vi "claustering trial 2.vi"() -> ()   [LabVIEW 2014]
panel:
  out "x = y?":bool[](array[boolean])
  out "Array 3":string[](array[string])
  out "logical AND":bool
  in  "how many clusters":i32
  in  "wf2":string[](array[string])=["0 3 0", "0 -2 0", "0 1 0", "0 3 -2", "2 -2 0", "0 2 0", "3 -2 0", "0 -3 4", "0 4 0", "-2 0 -2", "0 -3 0", "3 -2 2", "1 -1 0", "0 2 -2", "-2 3 -2", "0 -1 0", "0 -4 0", "0 2 -2 0", "-1 0 3", "0 -2 3", "2 0 -2", "0 3 -2 0", "0 -3 4 0", "-3 0 3", "0 3 -3", "4 -3 0", "-2 0 -3", "0 -2 3 -2", "-2 2 0", "0 3 -2 2", "3 -2 2 0", "2 0 2", "3 -3 0", "2 0 3", "0 -2 0 -2", "-3 4 0", "0 3 -3 0", "-1 0 3 0", "-2 0 1", "2 -1 0", "0 -3 4 -3", "0 3 -2 2 0", "-2 0 1 0", "-3 0 4", "0 -2 2", "-2 3 -2 0", "0 3 -2 3", "0 1 -1 0", "1 0 1", "0 -3 0 3", "0 -3 3", "3 0 -3", "0 -1 0 3", "4 0 1 0", "0 -2 3 -2 0", "2 0 3 -2 0", "0 2 -1", "3 -3 0 4 0", "-2 0 -4", "-3 0 -2", "3 0 3", "0 3 0 3 0", "0 3 -2 3 -2", "-2 3 -2 2", "-3 0 1", "-2 0 3", "-2 0 -3 0", "0 3 -2 2 0 2", "2 0 2 0", "1 -1 0 3", "0 3 -2 0 -2 2", "-2 0 -2 2", "2 0 -2 3 -2", "1 0 -2", "1 0 3", "2 0 -4 0", "-1 0 1", "0 2 0 4", "4 0 -2", "0 -2 0 1", "0 -1 0 3 0", "0 2 0 3 -2 0", "0 3 -2 0 1 0", "-1 0 -1 0", "-2 2 0 -2", "2 0 -2 0 -2", "0 4 0 1 0", "0 1 0 4 0", "0 1 0 -3", "0 -3 0 3 -2", "1 0 -3 0", "4 0 -4 0 1", "-1 0 -4", "0 -3 3 -3 0 4 0", "0 -4 0 3", "0 3 0 2", "1 0 1 0", "0 4 0 3", "1 -1 0 -3 4 0", "3 -2 0 -4", "2 -1 2 0", "-4 1 0", "3 -2 0 -4 0", "-2 0 -3 4", "0 -3 4 -3 0", "0 -2 0 -3", "-2 0 -3 4 -3 0", "2 -2 3", "0 2 -1 0", "2 0 2 -2 0", "0 -3 4 0 2", "1 0 2", "-3 4 0 2 0", "-2 0 -4 1", "0 3 -2 0 -4", "0 2 0 2", "-2 3 0", "1 0 -3", "0 3 0 -3 4", "-3 4 0 2", "-2 0 -2 2 -2 0", "2 -2 0 -3 4", "0 -3 4 -3 0 3", "4 -3 0 3 0", "3 0 -2", "0 -2 0 -2 0", "4 -3 0 3", "0 4 -3 0", "-3 0 -2 0", "-1 0 -1", "1 0 4", "2 0 2 -2", "-2 0 -2 0", "0 -1 0", "0 -2 3", "3 -2 0", "-2 3 -2 0", "0 2 0", "0 1 0", "0 4 0", "2 0 -1 0", "0 3 -2", "2 -2 3", "-2 0 2", "0 2 -2 0", "4 -3 0", "-3 0 -2 0", "0 3 0", "0 -3 -2", "-2 3 -2 0 3"]
  in  "wf1":string[](array[string])=["-2 2 0", "1 -1 0", "0 1 0", "0 -1 0", "3 -3 0", "0 3 0", "0 1 -1", "0 4 0", "0 2 0", "2 -1 0", "-1 0 1", "0 -2 0", "-4 1 0", "1 0 1", "0 1 -1 0", "-1 0 -3", "-1 0 4", "0 4 0 -2", "0 4 -4", "-1 0 1 0", "0 3 -3 0", "0 -4 1", "0 4 -4 1", "-4 4 0", "-1 0 3", "0 -2 3", "0 -3 4", "1 0 1 -1", "-2 0 -3", "0 -3 0", "0 -3 3", "-2 3 -3 0", "1 0 -2", "-2 3 -2", "4 -4 1", "1 -1 0 4 -4 1", "-1 0 4 -4 1 -1", "-4 1 0 1 -1 0", "0 1 0 -4", "0 1 0 -2", "-1 0 -1 0", "2 -1 0 1", "1 -1 0 1 0", "3 -2 0", "0 -2 2", "2 0 2", "3 -3 0 1", "-3 0 3", "-2 2 0 -3", "0 3 -3", "-3 0 -4 4", "0 4 0 -2 3", "0 -4 4", "-1 0 3 0", "4 -4 1 0 4", "4 0 1 0", "1 -1 0 -3", "-2 0 1 -1", "0 4 -4 1 0", "0 -4 4 0 1", "1 0 -2 3 -2", "1 0 4", "0 -4 1 0", "0 1 0 -4 1 0", "-2 0 1", "4 -3 0", "-3 0 4", "0 4 -3 0", "1 -1 0 4 -4 1 -1 0", "4 -4 1 0", "1 0 4 0", "1 -1 0 -1 0", "0 -4 0", "4 0 1", "0 1 0 1 0", "2 0 4 0", "0 -2 0 2 0", "2 0 1", "-1 0 -3 4", "4 0 2 0", "0 -2 0 1", "-1 0 4 -4 1", "3 -2 3", "3 -2 2 0", "1 -1 0 3", "-1 0 -1", "0 -1 1", "-1 0 1 0 3", "0 -4 1 0 1 -1 0", "0 3 -2", "0 1 0 3", "1 -4 0", "0 -2 2 0", "1 -1 1 -1 0", "0 1 0 3 -3 0", "-3 0 -3 3", "0 -3 3 0", "0 3 0 -2 0", "0 2 0 2", "-4 0 -2", "3 0 3", "3 0 3 0", "0 -3 3 -2", "0 2 -2 3 -3 0", "-2 2 0 -3 3", "-3 0 1", "3 -3 0 3", "0 3 -3 0 1", "0 3 0 2", "2 0 -3", "-2 3 -3", "3 -2 2", "-4 1 -1", "2 0 -3 3", "1 -1 0", "-1 0 1", "0 1 0", "0 -1 0", "0 1 -1", "-1 0 -1", "0 4 0", "2 -1 0", "-1 0 1 -1", "-1 0 4", "0 -3 0", "0 1 -1 0", "-1 1 -1", "-1 0 -3", "-1 0 -1 0", "0 -1 0 1", "1 -1 0 -1", "-1 1 -1 0", "1 -1 1", "4 0 2", "0 1 -1 0 1", "1 -1 0 4", "0 1 0 -4", "0 4 -4", "-1 0 -1 0 1", "-1 0 4 0", "0 1 -1 1 -1 0", "1 0 -4 0", "1 0 -4", "0 4 0 -1 0", "-1 0 1 0", "0 4 -4 0", "-1 0 -3 4 0", "0 1 0 -1 0 -3", "0 1 0 -4 0", "-4 0 4", "0 -1 1 -1", "-2 2 -1 0", "0 -3 0 -1 0", "2 -1 0 -3", "-1 0 3 0", "-1 0 -3 0", "-1 0 -2", "0 2 0", "1 -1 0 4 0", "-1 0 4 0 -1 0", "0 1 -1 1 -1 0 4", "0 -2 2 -2", "-1 0 -1 0 1 0", "3 0 1 0", "0 4 0 1 -1", "1 -1 0 1", "0 1 -1 1", "1 -1 1 -1", "0 1 -1 1 -1", "1 -1 1 -1 0", "0 -1 1", "0 -4 0", "-3 0 -1", "4 0 -1", "-1 1 -1 0 4", "1 -1 1 -1 0 4"]
  in  "jon1":string[](array[string])=["0 3 0", "0 1 0", "0 2 0", "0 4 0", "0 4 -4", "0 -3 4", "0 -3 0", "0 -4 0", "0 3 -2", "0 -1 0", "-4 1 0", "1 0 3", "0 2 0 -3", "2 0 3", "3 -3 0", "-3 0 3", "0 -3 3", "0 -3 4 -3 0", "0 -2 0", "3 -2 0", "0 3 0 1 0", "0 -3 4 0", "2 -2 0", "-2 0 -3", "4 0 2", "-3 0 2", "0 3 -3 0", "4 -4 0", "0 -1 2", "3 0 4", "0 3 -2 0", "0 -3 0 3", "1 0 -1", "0 4 -4 0", "-2 0 3", "0 2 -2 0", "0 2 0 -3 4", "3 -3 0 -3", "4 0 2 0", "3 0 -2", "0 -3 3 0", "-1 0 3", "0 -1 2 0", "-4 0 -1", "2 0 3 0", "0 3 0 3", "-4 0 3", "0 4 -4 1", "4 0 -3", "0 -1 0 4", "0 3 -3 0 2", "0 -2 0 3", "0 -3 4 0 3 0", "-3 0 4 0", "0 3 0 3 0", "0 4 0 -3 0", "-3 4 0", "2 0 -3 4", "0 2 0 -3 4 0", "0 1 0 2", "0 -2 3", "-2 0 -2", "0 -3 4 0 2", "0 -3 3 0 -2 2", "1 0 -3", "0 -1 1 0", "4 -4 0 -4", "-4 0 3 0", "2 0 -3", "-2 0 3 0", "0 4 -4 1 0", "-4 1 0 -1 2 0", "3 0 4 -4", "0 -3 4 -3 0 2", "3 0 3", "-1 0 -3", "-3 4 -3", "4 -3 0", "0 -3 4 -3", "-3 4 -3 0", "4 0 2 0 3", "0 2 0 3", "-4 1 0 -4 0 4 -4", "-4 1 -1", "-1 0 -4 0", "1 0 3 -2", "0 -1 0 3", "0 3 0 4 0", "0 2 0 3 0 1 0", "-4 1 -4 1", "1 -4 1 0", "0 -4 4", "0 1 0 4", "1 -4 1", "-3 0 1", "0 4 -4 0 -1 0", "-3 0 4", "2 0 -3 4 0", "1 0 2", "4 -3 0 2", "-3 4 -3 0 2", "3 0 1", "0 3 0", "0 -3 4", "0 -3 3", "0 3 -3 0", "0 2 0", "4 -3 0", "0 3 -3", "0 3 -2", "0 -3 4 -3 0", "-4 0 -3", "3 0 -3", "0 -4 0", "-3 0 -3", "0 -3 3 0 3", "0 -3 3 0", "0 -2 0", "-3 0 3", "3 -3 0", "3 0 3", "-3 4 0", "-4 0 -3 4", "-3 0 4", "0 -1 0", "3 0 -3 3", "-3 3 0", "0 3 -2 0", "0 -3 4 0", "1 0 -3 4", "0 -3 0", "0 -1 0 -3", "-3 0 3 0", "-2 0 3 -2", "0 1 0", "0 -2 0 3", "-2 0 -3", "0 3 0 -3", "3 0 3 -3", "3 -3 0 3", "-3 0 -3 3 0", "0 -3 4 -4 0", "0 2 0 -2", "-2 0 3", "0 3 -2 3 0", "-2 3 0 -3 3", "3 0 -1", "-3 0 -4", "1 -1 0", "-4 0 -2", "0 3 -3 0 4", "-2 3 0", "-1 0 3 -2", "-3 4 -3", "0 -3 4 -3", "-3 4 -3 0", "-3 3 0 3", "-2 0 2"]
  in  "jon2":string[](array[string])=["0 3 0", "0 -1 0", "0 4 0", "-1 0 3", "0 -3 4", "0 -3 3", "1 -1 0", "0 3 -2", "0 2 0", "0 1 -1", "4 -3 0", "-4 0 -3", "0 -4 0", "4 0 2", "0 1 -1 0", "0 1 0", "0 4 -4", "3 -2 2", "2 -1 0", "0 -2 0", "0 -3 4 0", "-1 0 -3", "0 3 -2 0", "0 -3 3 -3 0", "0 -3 4 -3 0", "4 0 4", "0 1 -1 0 3", "3 -2 2 0", "-2 2 0", "3 0 1", "0 4 0 2", "0 2 -1", "2 0 4", "-1 0 4", "0 -3 3 0", "-1 0 1", "-1 0 -1 0", "-1 0 -1", "4 -3 0 2", "0 -3 0", "-4 0 -3 0", "-3 0 3 -2", "0 3 -2 2 0", "-4 0 -3 3", "0 3 0 -4", "2 0 4 -4", "0 2 0 4", "0 4 0 -4", "2 -1 0 1 -1 0", "0 2 -1 0", "-1 0 -3 3", "0 -4 4 0", "0 4 -4 0", "-4 0 3 0", "0 -2 3", "-3 0 -3", "0 -2 0 -3", "-3 0 1", "-2 3 0", "0 3 0 -2", "0 4 -3 0", "4 -3 0 2 0", "0 -3 4 -3 0 3 -2 2 0", "3 0 -3 4 -3 0", "-1 0 3 -2 3", "-1 0 3 -2", "0 1 0 3", "1 0 3", "4 -3 0 -2", "-4 0 -3 4", "-2 0 3 0", "2 0 2", "0 2 0 2 0", "-4 4 -3 0", "0 -4 0 -3", "3 0 3 0", "-4 0 -3 3 0", "4 0 3", "0 4 0 4", "4 0 4 0", "0 4 0 -4 0", "0 -1 0 -2", "4 0 2 0", "1 0 -3", "0 -4 1 -4", "0 4 -4 0 -3", "-2 2 0 4 -4", "0 4 -4 4 -4", "4 0 2 -2", "0 4 0 -2", "0 3 0 1", "4 -4 1", "4 0 2 -1 0", "0 -4 4 0 2", "-1 0 3 0", "0 3 -2 0 -1 0", "1 -1 0 4", "0 4 0 1", "-1 0 4 0", "1 0 3 -2 0 -1 0", "0 -4 0 3 0 -4", "-1 0 -4", "1 -4 0", "1 0 4 0", "0 -1 0 -1 0", "-1 0 -3 3 0", "0 -1 0 -1 0 -3", "-2 2 -1 0", "0 -1 0 3 -2", "2 -1 0 1 -1 0 3", "-2 3 -2 2 -1", "-2 2 -1", "0 -1 0 4", "3 0 1 0", "0 3 -2 0 -1 0 -1 0", "-3 4 0", "3 0 -1", "0 4 -3", "3 0 3", "-4 0 3", "4 -4 0", "0 -1 0 -1", "1 -1 0", "0 -1 0", "0 1 0", "0 1 -1 0", "0 4 0", "0 3 0", "-1 0 4", "-1 0 -3 3", "1 0 1", "-4 1 -1", "0 4 0 2", "0 -1 0 -3", "3 -2 2 -1 0", "2 -1 0", "0 1 -1", "-1 0 3", "-1 1 -1 0", "-3 0 1", "-1 0 3 0 -4", "-1 0 -3", "1 -1 0 -3 3", "1 -1 0 3", "2 -1 0 4 -4", "1 0 1 0", "0 -1 0 4", "2 0 3 0 -1", "-4 1 -1 0"]
  in  "CSS validated and checked":string[](array[string])=["0 1 0", "0 -1 0", "0 2 0", "0 4 0", "-4 1 0", "0 -4 0", "0 -2 0", "1 0 4", "1 -4 0", "0 -3 3", "0 -3 0", "1 -1 0", "-2 2 0", "0 1 -4", "2 0 -3", "0 -3 3 0", "-1 0 -1", "0 -1 1", "2 -1 0", "0 2 -1", "-3 0 1", "0 1 0 4", "1 0 4 0", "-3 3 0", "1 0 -3", "3 -2 0", "2 0 -3 0", "1 0 -1", "-4 0 -1", "0 -4 1", "2 0 -1", "0 -2 2", "-4 0 -3", "0 -1 1 0", "0 2 0 -3", "3 -3 0", "-4 0 1 0", "-4 1 -4 0", "-4 1 0 4", "0 1 -4 0", "-4 1 -4", "0 2 -1 0", "1 0 3", "0 -3 4 0", "-2 0 2", "1 0 1", "4 0 2 0", "0 2 0 3", "0 -1 2", "-1 0 -4", "1 0 -4", "0 -1 0 -1", "-1 0 2", "-1 0 -1 0", "1 0 -2", "0 -4 0 -1", "0 -2 2 0", "-1 0 1", "2 0 2", "0 1 -1 0", "0 3 -3 0", "-4 0 -2", "0 4 -4", "0 -4 0 -3", "0 4 0 1", "0 -2 0 2", "0 4 0 2 0", "-3 0 1 -4 0 -3", "2 0 1 0", "-2 0 2 0", "0 3 -2 0", "-3 3 0 -2 0", "3 -3 0 1", "-3 0 1 0", "4 -4 0", "0 4 -4 0", "0 -3 3 0 -2", "2 0 2 0", "-2 0 -1", "0 -4 0 1 0", "2 0 -4 0", "2 0 -1 0", "-1 3 -2", "2 0 1", "1 0 -3 3 0", "-4 1 -1", "-4 1 -1 0", "-1 0 -3", "3 -2 2", "-1 1 -1 0", "2 0 4", "1 0 -1 0", "0 -1 2 -1", "0 2 0 -2", "-3 0 -4 1", "0 1 0 -1", "-1 3 0", "0 -1 0 -4", "-2 0 -1 0", "4 0 4", "-4 1 0 4 0", "-4 0 -2 0", "-4 0 2", "0 -2 0 2 0", "0 2 0 -4 0", "2 0 4 0", "4 0 -2", "0 1 0 -4 0", "3 0 1", "2 -2 0", "4 0 -2 0", "0 2 0 4", "1 -4 0 1 0", "0 2 0 -2 0", "-2 2 0 -1 0", "-2 2 0 -1", "-1 0 4 0", "-2 0 4", "-4 1 0 3", "0 -3 0 1", "-2 2 0 -3 0", "0 1 0 3", "0 2 0 1", "0 1 0 1 -4", "0 1 -4 1", "-4 1 0 -3", "1 0 -3 0", "-3 0 -2", "2 -1 0 -1 0", "-3 3 0 -2", "1 0 4 -4 0", "0 -4 0 -3 0", "0 -4 0 1 0 -3 3 0", "0 -3 3 0 2 0 -3 0", "0 -3 3 -3 0", "3 -2 0 1", "-4 0 3", "-2 0 1", "0 3 0", "0 -3 4", "-3 4 0", "-3 0 4", "0 3 -3 0 1 -4 0 -3 3", "0 -2 0 -1", "-4 1 0 -2", "-4 0 -2 0 -1", "-2 0 -4", "0 1 0 -2", "0 -1 0 2 0", "0 -2 2 0 -1", "0 -3 -1 3", "-4 -1 0", "0 -1 2 0", "0 -3 0 -4", "2 0 -3 0 -4", "3 0 -1 1", "-4 1 0 -1", "-1 0 -1 2", "-1 0 -4 0", "0 -4 1 -1", "-3 3 -2", "2 -1 1", "4 -3 0", "1 -4 4", "0 2 0 -1", "1 0 1 0", "4 1 0", "0 2 0 2 0", "-4 0 -1 -3", "1 -4 0 -1", "0 -4 1 -4", "-1 3 0 -4 1 -4", "2 -1 3", "1 -3 0", "-2 0 1 -4", "1 0 -1 1", "0 -3 0 -4 1", "0 2 -1 0 1 -4", "0 -1 3", "0 -4 0 -1 0", "0 4 0 -2", "0 -2 0 -1 0", "0 -3 3 0 -2 0", "0 1 -1 0 -1", "0 -1 0 1 -1 0", "-1 3 -2 2", "-2 2 0 1 0 -1", "0 1 -1", "0 4 0 1 0 4", "-3 0 -4", "1 0 4 0 4 0", "4 -4 0 -2", "4 0 2", "-1 2 0", "1 -1 0 -1", "4 0 1", "2 0 3", "0 2 0", "0 -1 0", "0 1 0", "0 3 0", "0 -4 0", "-2 2 0", "1 -1 0", "0 -2 0", "0 -1 2", "0 1 -1", "0 3 -2", "3 -2 0", "0 2 -2", "-1 0 3", "2 -1 0", "-1 0 -1", "-1 0 -3", "-2 2 -2", "2 0 1", "2 0 2", "0 -3 0", "3 -2 2", "0 1 -1 0", "0 -2 2", "-1 2 0", "2 0 -1", "2 -2 0", "3 -3 0", "0 -1 2 0", "0 -1 0 3", "0 -1 1", "0 2 0 1", "2 -2 2", "0 -4 4", "0 4 0", "2 0 3", "-2 3 -2", "2 -2 3", "4 -4 0", "0 1 0 -3", "0 3 0 3", "-1 0 4", "-3 0 -2", "-4 0 -2", "2 0 2 -1", "-1 0 2", "-2 0 -1", "-4 4 0", "0 2 0 -2", "-1 1 -1", "-1 1 -1 0", "-2 0 -2", "3 0 -4 0", "3 0 3", "0 1 0 3", "0 3 -3 0", "2 0 -2", "3 0 -2", "0 -3 3", "3 -2 2 -2", "-3 0 -2 0", "1 0 -3 0", "-1 0 2 0", "3 0 -4", "-1 0 1", "-1 0 -1 0", "0 -1 2 3", "-1 3 -2 0", "3 -1 3", "-2 0 2 0", "0 1 0 -3 0", "0 -4 0 -2", "1 4 -4", "0 -2 2 0", "1 4 0", "0 3 -2 0", "-2 0 -4 4", "-1 0 3 0", "0 2 0 -1", "0 2 -2 3", "4 0 -1", "-1 2 0 2", "1 -1 0 -3", "-2 0 2", "2 0 -4", "0 3 -2 2 -2 2", "0 2 -2 0", "4 0 -4 0", "0 3 0 3 0", "4 -3 0", "-3 4 -3 0", "0 4 -4", "3 0 -1", "-2 2 -2 0", "0 -2 3", "-2 0 3", "1 0 -3", "2 -2 2 0", "0 -3 4", "0 -1 1 -1", "0 4 1 4", "1 -1 0 -1", "1 4 -4 0", "-4 0 2 0", "-4 0 2", "0 -2 2 3 0", "0 -1 1 -1 0", "0 2 0 1 4", "4 0 1 0", "2 3 -2", "0 -1 2 3 -2", "0 -1 0 4", "-4 0 1", "-1 0 -1 2", "-2 0 -1 0", "0 3 0 -1", "3 -2 0 -1", "0 -4 0 -2 0", "2 0 -4 0", "0 -2 0 2", "-1 0 -3 0", "0 -3 0 -2", "2 0 -1 0", "0 -1 2 0 1", "0 -2 0 -4 4 0", "0 -4 4 0", "-1 -3 0", "0 -2 0 3", "2 0 -2 2", "-4 1 0", "-1 1 4", "-1 0 3 -2", "0 2 0 4", "0 -4 4 0 -1", "3 0 -2 0", "0 3 0 -2", "2 0 1 -1 0", "0 1 -1 0 2 0", "0 2 0 1 -1", "2 0 -1 2", "-2 3 0", "0 -1 0 2", "0 1 -1 0 -3", "2 0 1 -1", "-2 0 -1 2", "-1 4 0", "0 -4 1", "2 0 2 0", "2 -1 1", "4 -4 0 -1", "-4 0 -1", "-1 0 4 0", "2 0 2 -1 0", "0 -3 3 0", "-1 0 -3 3", "-1 0 1 -1 0", "0 3 0 -4", "-2 2 -2 0 -2", "-2 0 4 0", "0 1 0 3 0", "4 -3 0 -2 0", "0 3 -2 3", "2 0 3 -2", "3 -2 3", "0 2 -2 3 -2 2", "-2 2 0 3", "3 -2 2 0", "3 -2 2 0 3", "3 -2 3 -2", "0 -3 4 -3 0", "0 -1 0 -3", "3 -3 0 1 0", "0 2 0 3", "0 3 -2 2 -2 2 0", "0 2 0 2", "-2 3 -2 0", "4 0 -2", "-4 0 -1 0 3", "-2 2 -2 3", "0 -1 0 -1 0", "-2 2 0 3 0", "0 2 -2 2", "2 3 -2 2 0", "-2 2 -1", "-4 0 -2 2", "0 -4 0 2", "-1 2 -1", "-1 0 3 -1 3 0 -4", "-1 3 -2", "4 0 -4", "3 0 3 0", "0 3 0", "0 1 0", "0 2 0", "0 4 0", "0 4 -4", "0 -3 4", "0 -3 0", "0 -4 0", "0 3 -2", "0 -1 0", "-4 1 0", "1 0 3", "0 2 0 -3", "2 0 3", "3 -3 0", "-3 0 3", "0 -3 3", "0 -3 4 -3 0", "0 -2 0", "3 -2 0", "0 3 0 1 0", "0 -3 4 0", "2 -2 0", "-2 0 -3", "4 0 2", "-3 0 2", "0 3 -3 0", "4 -4 0", "0 -1 2", "3 0 4", "0 3 -2 0", "0 -3 0 3", "1 0 -1", "0 4 -4 0", "-2 0 3", "0 2 -2 0", "0 2 0 -3 4", "3 -3 0 -3", "4 0 2 0", "3 0 -2", "0 -3 3 0", "-1 0 3", "0 -1 2 0", "-4 0 -1", "2 0 3 0", "0 3 0 3", "-4 0 3", "0 4 -4 1", "4 0 -3", "0 -1 0 4", "0 3 -3 0 2", "0 -2 0 3", "0 -3 4 0 3 0", "-3 0 4 0", "0 3 0 3 0", "0 4 0 -3 0", "-3 4 0", "2 0 -3 4", "0 2 0 -3 4 0", "0 1 0 2", "0 -2 3", "-2 0 -2", "0 -3 4 0 2", "0 -3 3 0 -2 2", "1 0 -3", "0 -1 1 0", "4 -4 0 -4", "-4 0 3 0", "2 0 -3", "-2 0 3 0", "0 4 -4 1 0", "-4 1 0 -1 2 0", "3 0 4 -4", "0 -3 4 -3 0 2", "3 0 3", "-1 0 -3", "-3 4 -3", "4 -3 0", "0 -3 4 -3", "-3 4 -3 0", "4 0 2 0 3", "0 2 0 3", "-4 1 0 -4 0 4 -4", "-4 1 -1", "-1 0 -4 0", "1 0 3 -2", "0 -1 0 3", "0 3 0 4 0", "0 2 0 3 0 1 0", "-4 1 -4 1", "1 -4 1 0", "0 -4 4", "0 1 0 4", "1 -4 1", "-3 0 1", "0 4 -4 0 -1 0", "-3 0 4", "2 0 -3 4 0", "1 0 2", "4 -3 0 2", "-3 4 -3 0 2", "3 0 1", "1 -1 0", "0 -1 0", "0 1 0", "0 1 -1 0", "0 4 0", "0 3 0", "-1 0 4", "-1 0 -3 3", "1 0 1", "-4 1 -1", "0 4 0 2", "0 -1 0 -3", "3 -2 2 -1 0", "2 -1 0", "0 1 -1", "-1 0 3", "-1 1 -1 0", "-3 0 1", "-1 0 3 0 -4", "-1 0 -3", "1 -1 0 -3 3", "1 -1 0 3", "2 -1 0 4 -4", "1 0 1 0", "0 -1 0 4", "2 0 3 0 -1", "-4 1 -1 0", "0 3 0", "0 -1 0", "0 4 0", "-1 0 3", "0 -3 4", "0 -3 3", "1 -1 0", "0 3 -2", "0 2 0", "0 1 -1", "4 -3 0", "-4 0 -3", "0 -4 0", "4 0 2", "0 1 -1 0", "0 1 0", "0 4 -4", "3 -2 2", "2 -1 0", "0 -2 0", "0 -3 4 0", "-1 0 -3", "0 3 -2 0", "0 -3 3 -3 0", "0 -3 4 -3 0", "4 0 4", "0 1 -1 0 3", "3 -2 2 0", "-2 2 0", "3 0 1", "0 4 0 2", "0 2 -1", "2 0 4", "-1 0 4", "0 -3 3 0", "-1 0 1", "-1 0 -1 0", "-1 0 -1", "4 -3 0 2", "0 -3 0", "-4 0 -3 0", "-3 0 3 -2", "0 3 -2 2 0", "-4 0 -3 3", "0 3 0 -4", "2 0 4 -4", "0 2 0 4", "0 4 0 -4", "2 -1 0 1 -1 0", "0 2 -1 0", "-1 0 -3 3", "0 -4 4 0", "0 4 -4 0", "-4 0 3 0", "0 -2 3", "-3 0 -3", "0 -2 0 -3", "-3 0 1", "-2 3 0", "0 3 0 -2", "0 4 -3 0", "4 -3 0 2 0", "0 -3 4 -3 0 3 -2 2 0", "3 0 -3 4 -3 0", "-1 0 3 -2 3", "-1 0 3 -2", "0 1 0 3", "1 0 3", "4 -3 0 -2", "-4 0 -3 4", "-2 0 3 0", "2 0 2", "0 2 0 2 0", "-4 4 -3 0", "0 -4 0 -3", "3 0 3 0", "-4 0 -3 3 0", "4 0 3", "0 4 0 4", "4 0 4 0", "0 4 0 -4 0", "0 -1 0 -2", "4 0 2 0", "1 0 -3", "0 -4 1 -4", "0 4 -4 0 -3", "-2 2 0 4 -4", "0 4 -4 4 -4", "4 0 2 -2", "0 4 0 -2", "0 3 0 1", "4 -4 1", "4 0 2 -1 0", "0 -4 4 0 2", "-1 0 3 0", "0 3 -2 0 -1 0", "1 -1 0 4", "0 4 0 1", "-1 0 4 0", "1 0 3 -2 0 -1 0", "0 -4 0 3 0 -4", "-1 0 -4", "1 -4 0", "1 0 4 0", "0 -1 0 -1 0", "-1 0 -3 3 0", "0 -1 0 -1 0 -3", "-2 2 -1 0", "0 -1 0 3 -2", "2 -1 0 1 -1 0 3", "-2 3 -2 2 -1", "-2 2 -1", "0 -1 0 4", "3 0 1 0", "0 3 -2 0 -1 0 -1 0", "-3 4 0", "3 0 -1", "0 4 -3", "3 0 3", "-4 0 3", "4 -4 0", "0 -1 0 -1", "0 3 0", "0 -3 4", "0 -3 3", "0 3 -3 0", "0 2 0", "4 -3 0", "0 3 -3", "0 3 -2", "0 -3 4 -3 0", "-4 0 -3", "3 0 -3", "0 -4 0", "-3 0 -3", "0 -3 3 0 3", "0 -3 3 0", "0 -2 0", "-3 0 3", "3 -3 0", "3 0 3", "-3 4 0", "-4 0 -3 4", "-3 0 4", "0 -1 0", "3 0 -3 3", "-3 3 0", "0 3 -2 0", "0 -3 4 0", "1 0 -3 4", "0 -3 0", "0 -1 0 -3", "-3 0 3 0", "-2 0 3 -2", "0 1 0", "0 -2 0 3", "-2 0 -3", "0 3 0 -3", "3 0 3 -3", "3 -3 0 3", "-3 0 -3 3 0", "0 -3 4 -4 0", "0 2 0 -2", "-2 0 3", "0 3 -2 3 0", "-2 3 0 -3 3", "3 0 -1", "-3 0 -4", "1 -1 0", "-4 0 -2", "0 3 -3 0 4", "-2 3 0", "-1 0 3 -2", "-3 4 -3", "0 -3 4 -3", "-3 4 -3 0", "-3 3 0 3", "-2 0 2", "0 -1 0", "0 -2 3", "3 -2 0", "-2 3 -2 0", "0 2 0", "0 1 0", "0 4 0", "2 0 -1 0", "0 3 -2", "2 -2 3", "-2 0 2", "0 2 -2 0", "4 -3 0", "-3 0 -2 0", "0 3 0", "0 -3 -2", "-2 3 -2 0 3", "0 3 0", "0 -2 0", "0 1 0", "0 3 -2", "2 -2 0", "0 2 0", "3 -2 0", "0 -3 4", "0 4 0", "-2 0 -2", "0 -3 0", "3 -2 2", "1 -1 0", "0 2 -2", "-2 3 -2", "0 -1 0", "0 -4 0", "0 2 -2 0", "-1 0 3", "0 -2 3", "2 0 -2", "0 3 -2 0", "0 -3 4 0", "-3 0 3", "0 3 -3", "4 -3 0", "-2 0 -3", "0 -2 3 -2", "-2 2 0", "0 3 -2 2", "3 -2 2 0", "2 0 2", "3 -3 0", "2 0 3", "0 -2 0 -2", "-3 4 0", "0 3 -3 0", "-1 0 3 0", "-2 0 1", "2 -1 0", "0 -3 4 -3", "0 3 -2 2 0", "-2 0 1 0", "-3 0 4", "0 -2 2", "-2 3 -2 0", "0 3 -2 3", "0 1 -1 0", "1 0 1", "0 -3 0 3", "0 -3 3", "3 0 -3", "0 -1 0 3", "4 0 1 0", "0 -2 3 -2 0", "2 0 3 -2 0", "0 2 -1", "3 -3 0 4 0", "-2 0 -4", "-3 0 -2", "3 0 3", "0 3 0 3 0", "0 3 -2 3 -2", "-2 3 -2 2", "-3 0 1", "-2 0 3", "-2 0 -3 0", "0 3 -2 2 0 2", "2 0 2 0", "1 -1 0 3", "0 3 -2 0 -2 2", "-2 0 -2 2", "2 0 -2 3 -2", "1 0 -2", "1 0 3", "2 0 -4 0", "-1 0 1", "0 2 0 4", "4 0 -2", "0 -2 0 1", "0 -1 0 3 0", "0 2 0 3 -2 0", "0 3 -2 0 1 0", "-1 0 -1 0", "-2 2 0 -2", "2 0 -2 0 -2", "0 4 0 1 0", "0 1 0 4 0", "0 1 0 -3", "0 -3 0 3 -2", "1 0 -3 0", "4 0 -4 0 1", "-1 0 -4", "0 -3 3 -3 0 4 0", "0 -4 0 3", "0 3 0 2", "1 0 1 0", "0 4 0 3", "1 -1 0 -3 4 0", "3 -2 0 -4", "2 -1 2 0", "-4 1 0", "3 -2 0 -4 0", "-2 0 -3 4", "0 -3 4 -3 0", "0 -2 0 -3", "-2 0 -3 4 -3 0", "2 -2 3", "0 2 -1 0", "2 0 2 -2 0", "0 -3 4 0 2", "1 0 2", "-3 4 0 2 0", "-2 0 -4 1", "0 3 -2 0 -4", "0 2 0 2", "-2 3 0", "1 0 -3", "0 3 0 -3 4", "-3 4 0 2", "-2 0 -2 2 -2 0", "2 -2 0 -3 4", "0 -3 4 -3 0 3", "4 -3 0 3 0", "3 0 -2", "0 -2 0 -2 0", "4 -3 0 3", "0 4 -3 0", "-3 0 -2 0", "-1 0 -1", "1 0 4", "2 0 2 -2", "-2 0 -2 0", "1 -1 0", "-1 0 1", "0 1 0", "0 -1 0", "0 1 -1", "-1 0 -1", "0 4 0", "2 -1 0", "-1 0 1 -1", "-1 0 4", "0 -3 0", "0 1 -1 0", "-1 1 -1", "-1 0 -3", "-1 0 -1 0", "0 -1 0 1", "1 -1 0 -1", "-1 1 -1 0", "1 -1 1", "4 0 2", "0 1 -1 0 1", "1 -1 0 4", "0 1 0 -4", "0 4 -4", "-1 0 -1 0 1", "-1 0 4 0", "0 1 -1 1 -1 0", "1 0 -4 0", "1 0 -4", "0 4 0 -1 0", "-1 0 1 0", "0 4 -4 0", "-1 0 -3 4 0", "0 1 0 -1 0 -3", "0 1 0 -4 0", "-4 0 4", "0 -1 1 -1", "-2 2 -1 0", "0 -3 0 -1 0", "2 -1 0 -3", "-1 0 3 0", "-1 0 -3 0", "-1 0 -2", "0 2 0", "1 -1 0 4 0", "-1 0 4 0 -1 0", "0 1 -1 1 -1 0 4", "0 -2 2 -2", "-1 0 -1 0 1 0", "3 0 1 0", "0 4 0 1 -1", "1 -1 0 1", "0 1 -1 1", "1 -1 1 -1", "0 1 -1 1 -1", "1 -1 1 -1 0", "0 -1 1", "0 -4 0", "-3 0 -1", "4 0 -1", "-1 1 -1 0 4", "1 -1 1 -1 0 4", "-2 2 0", "1 -1 0", "0 1 0", "0 -1 0", "3 -3 0", "0 3 0", "0 1 -1", "0 4 0", "0 2 0", "2 -1 0", "-1 0 1", "0 -2 0", "-4 1 0", "1 0 1", "0 1 -1 0", "-1 0 -3", "-1 0 4", "0 4 0 -2", "0 4 -4", "-1 0 1 0", "0 3 -3 0", "0 -4 1", "0 4 -4 1", "-4 4 0", "-1 0 3", "0 -2 3", "0 -3 4", "1 0 1 -1", "-2 0 -3", "0 -3 0", "0 -3 3", "-2 3 -3 0", "1 0 -2", "-2 3 -2", "4 -4 1", "1 -1 0 4 -4 1", "-1 0 4 -4 1 -1", "-4 1 0 1 -1 0", "0 1 0 -4", "0 1 0 -2", "-1 0 -1 0", "2 -1 0 1", "1 -1 0 1 0", "3 -2 0", "0 -2 2", "2 0 2", "3 -3 0 1", "-3 0 3", "-2 2 0 -3", "0 3 -3", "-3 0 -4 4", "0 4 0 -2 3", "0 -4 4", "-1 0 3 0", "4 -4 1 0 4", "4 0 1 0", "1 -1 0 -3", "-2 0 1 -1", "0 4 -4 1 0", "0 -4 4 0 1", "1 0 -2 3 -2", "1 0 4", "0 -4 1 0", "0 1 0 -4 1 0", "-2 0 1", "4 -3 0", "-3 0 4", "0 4 -3 0", "1 -1 0 4 -4 1 -1 0", "4 -4 1 0", "1 0 4 0", "1 -1 0 -1 0", "0 -4 0", "4 0 1", "0 1 0 1 0", "2 0 4 0", "0 -2 0 2 0", "2 0 1", "-1 0 -3 4", "4 0 2 0", "0 -2 0 1", "-1 0 4 -4 1", "3 -2 3", "3 -2 2 0", "1 -1 0 3", "-1 0 -1", "0 -1 1", "-1 0 1 0 3", "0 -4 1 0 1 -1 0", "0 3 -2", "0 1 0 3", "1 -4 0", "0 -2 2 0", "1 -1 1 -1 0", "0 1 0 3 -3 0", "-3 0 -3 3", "0 -3 3 0", "0 3 0 -2 0", "0 2 0 2", "-4 0 -2", "3 0 3", "3 0 3 0", "0 -3 3 -2", "0 2 -2 3 -3 0", "-2 2 0 -3 3", "-3 0 1", "3 -3 0 3", "0 3 -3 0 1", "0 3 0 2", "2 0 -3", "-2 3 -3", "3 -2 2", "-4 1 -1", "2 0 -3 3", "0 4 0", "0 -2 0", "1 -1 0", "-1 2 -1", "0 2 0", "2 -1 0", "0 3 0", "0 -1 0", "-2 0 3", "0 -4 0", "3 -2 0", "0 3 -2", "0 -3 0", "-1 0 3", "0 -2 0 3", "0 1 -1 0", "0 3 -2 0", "1 -4 0", "-1 0 2", "0 -1 2", "2 0 3", "0 -3 3", "3 -3 0", "3 0 -1 0", "-2 0 -2", "2 -2 0", "-3 3 0", "0 2 0 3", "0 1 0", "0 -2 2", "-4 0 -1", "0 -1 2 -1", "-1 0 -1", "2 -1 2", "-1 3 -2", "3 0 -4", "3 -2 2", "-1 1 -1 0", "-1 2 -1 0", "0 1 -4", "4 -4 0", "2 -3 0", "0 3 0 -2", "2 0 3 0", "0 1 0 -3", "1 0 -3", "-1 0 -4 0", "-4 0 1", "2 0 -2 0", "-1 0 -3", "0 -3 4", "4 0 1", "0 1 -4 0", "0 -1 0 3", "0 -3 3 0", "0 3 -3 0", "0 4 0 2", "0 2 -2 0", "-2 0 -3", "3 0 3", "-1 0 -2", "-2 0 3 0", "2 0 4 0", "0 4 0 -2 3", "0 -3 0 -2", "-3 0 -2 2", "1 0 4 0", "-3 0 2", "0 -2 0 3 -2 0", "1 0 -3 0", "-3 0 -2", "-2 0 -2 0", "0 4 -4", "-1 -3 0", "-2 2 -1", "2 0 -3", "-1 1 0", "2 -1 1", "-2 2 0", "0 -4 0 -1", "0 -1 3 -2 2", "-1 2 -1 2", "-1 2 0", "-1 3 0 -1 0", "2 0 2", "-1 0 2 -3 0", "-1 0 2 0", "-1 4 -4 1", "-1 0 4", "2 -1 0 -1", "2 -1 0 2", "-4 1 -1", "3 0 -4 1", "1 -1 -3 3", "0 1 0", "0 -2 0", "1 -1 0", "0 3 0", "0 2 0", "0 3 -2", "3 -2 0", "0 -4 0", "-1 0 -2", "-2 2 0", "0 -1 0", "1 -1 0 -2", "0 -2 2", "-2 0 -2", "0 1 0 1", "4 -4 0", "0 3 -3", "0 1 -1", "1 0 1", "0 3 -2 0", "-2 2 -2", "0 -2 3", "0 3 -3 0", "0 4 0", "2 0 3", "0 -2 3 -2", "0 4 -4 0", "-2 0 -2 0", "1 -1 0 -2 0", "-2 0 2", "-4 0 -4", "0 -4 0 1", "0 2 0 -4", "3 0 -2", "-1 0 3", "0 1 -1 0", "-3 0 -1", "-1 0 2 0", "4 -3 0", "1 0 -2", "0 1 0 1 0", "0 -2 3 -2 0", "3 -2 0 -2 0", "0 -2 2 -2 0", "0 -2 0 -2", "-1 4 0", "4 0 2", "1 -1 0 -2 0 2 0", "2 0 -2", "-2 0 4", "0 -1 0 3", "0 -2 2 0", "1 0 3", "0 1 0 3", "4 0 -2", "0 -4 0 -4", "0 2 0 -4 0", "-4 0 -4 0 1 0", "-1 2 3 0", "3 0 3", "0 -4 0 3 0", "2 0 1", "2 -1 0", "-1 0 -1", "-2 3 0 -2", "3 0 -2 0", "0 1 -1 0 -2", "0 3 0 -2", "3 -2 2 -2", "1 0 1 -1", "0 4 -3 0", "2 0 -1 0", "0 2 0 3", "2 0 3 0", "2 0 -3 4 -3", "-2 2 0 -3 4", "2 0 -3 4", "0 3 -3 0 -1 0", "1 0 4", "0 3 0 1", "1 0 3 -2 0", "-2 3 0", "1 0 1 0", "0 4 0", "0 2 0", "0 3 0", "0 -3 0", "0 1 0", "-4 0 -3", "0 -4 0", "0 3 -3 0", "0 -3 0 3", "-4 0 3", "0 4 0 2", "0 -3 3", "-4 0 -3 0 3", "0 2 0 3", "-3 0 2", "0 4 0 1", "0 -4 0 3", "0 4 0 2 0", "0 -2 0", "0 1 0 4", "4 0 2", "0 4 0", "0 3 0", "0 2 0", "4 -4 0", "0 4 -4 0", "0 -2 0", "3 -3 0", "0 4 -4", "0 3 -3", "0 3 -2", "0 4 0 2", "4 0 2", "0 1 0", "0 3 -3 0", "0 -3 0", "2 -1 0", "0 -1 0", "1 0 3", "4 0 3", "3 -2 0", "0 1 -4", "-1 0 4", "0 -4 0", "0 -3 3", "2 0 4", "-4 1 0", "0 -2 2", "0 4 0 3", "-1 0 1", "0 3 -2 0", "-3 0 4", "-1 0 3", "0 -3 4", "0 4 0 -2", "1 -1 0", "2 0 4 0", "0 -4 4", "0 -1 0 4", "-1 0 4 0", "4 -3 0", "0 2 -1 0", "1 -4 0", "2 0 -4", "-2 0 4", "0 4 0 2 0", "3 0 3", "0 -3 3 0", "2 -2 0", "1 0 -3", "-4 0 2", "1 0 3 0", "0 1 0 3", "-1 0 3 0", "3 -2 2", "-4 1 -1", "2 0 -3", "0 -4 1", "0 2 0 -4", "-3 0 4 0", "3 0 -2", "0 -2 2 0", "0 -2 3", "-4 0 2 0", "0 3 0 -4", "0 2 0 4 0", "-2 0 2", "-2 2 0", "0 3 0 4", "-3 4 0", "-1 0 1 0", "4 0 4", "0 1 0 3 0", "0 -1 0 4 0", "0 3 0 3", "1 0 -3 0", "0 3 0 1", "-2 2 -1 0", "0 3 -2 2", "-3 0 2", "1 -1 0 3 0", "0 3 0 -2", "-4 0 -4", "0 1 0 -3 0", "0 4 0 -3", "2 -1 0 4", "1 -4 1", "-4 0 3", "-2 0 -4 0", "0 3 -3 0 4", "-4 0 -2", "0 4 -4 0 3", "0 -2 3 -2 0", "0 4 0 4", "-1 2 -1", "-3 0 -2", "-3 0 -3", "-4 0 4", "4 0 -3", "3 0 -4", "2 0 -2", "-2 0 2 0", "0 -4 4 0", "0 2 0 3", "-2 0 1", "4 0 3 -3 0", "0 -2 0 3", "0 4 0 3 0", "0 2 -2 0", "2 -2 0 4", "4 0 -2", "2 0 -1", "0 1 -4 0", "0 -1 2", "4 0 -1", "0 1 -4 1", "4 -4 1", "0 3 -2 0 1", "4 0 4 0", "0 -1 0 4 0 4", "1 0 4", "0 1 -4 1 0", "0 4 0 2 0 -3", "-2 0 4 0", "0 2 -2 0 4 0", "0 -3 0 2", "-4 0 -2 0", "0 -2 0 2 0", "0 2 0 -1", "0 -1 3", "0 -4 4 -4", "3 -2 0 -4 0", "-4 0 -1", "-3 0 3 0 3", "-1 0 3 -3 0", "-3 0 3 0", "0 3 0 3 -2", "-2 2 -2", "-1 0 1 0 3", "-2 2 -1 0 1 0", "0 2 -1 0 -3", "0 4 0 2 -1 0", "-1 0 4 -4 0", "0 2 -1 0 4 -4", "0 4 -4 0 3 -2 0", "-1 0 -3", "-2 0 1 -4", "0 3 0 4 0", "0 1 -4 4", "-1 0 -3 0", "-1 0 4 -4", "0 4 0 -2 0", "0 4 -3 0", "4 0 -3 3", "-1 0 -2", "0 -2 0 3 -3", "1 -4 1 -1 0", "-4 1 -1 0", "-2 0 -2 2", "0 -1 2 -1", "-4 0 -4 1", "0 2 0 4 0 2 0", "0 3 0 -1", "3 0 3 0", "0 -3 0 3 0", "0 3 0 4 -4 1", "-1 0 -4", "0 -4 1 0 3 0", "0 2 -1", "-4 0 4 0", "0 -2 0 4", "0 4 0 -1", "-4 0 3 0", "0 3 0 -2 0", "0 -3 4 -3 0", "-4 0 2 0 -4", "2 0 -2 0", "-2 2 0 -3", "3 0 2 0 4 0", "3 0 2 0", "1 -4 0 2 0", "3 0 -4 4 0", "3 0 -4 4", "3 -3 0 4", "-2 3 -3", "0 -4 0 2 0", "0 3 0 -4 0", "3 -3 0 4 0", "0 3 -3 0 4 0", "4 0 3 -2", "-4 0 -3", "-3 0 -3 4", "3 -3 4 0", "1 -4 -1", "-3 3 -3 0", "0 -1 1", "-3 0 4 0 3", "0 3 -3 0 -2", "0 4 0 3 -3 0", "4 -3 0 4", "0 3 0 2 0", "0 4 0 -2 2", "-4 -1 0 1", "-1 0 1 0 -3 0", "-3 0 1 -4 0", "-3 3 0", "0 -1 0 1", "-1 0 1 -4", "0 3 0 -4 4", "-4 1 -1 0 3 0", "0 1 0 3 0 1", "-3 0 3", "4 0 -2 0", "4 0 2 0", "3 0 -1", "4 0 3 -3", "3 -3 0 -2", "3 0 4", "3 0 2", "2 0 3", "4 0 -2 2", "-2 2 -1", "0 2 -1", "0 4 0", "2 -1 0", "0 -4 0", "0 2 -1 0", "3 -2 0", "4 -3 0", "0 -1 2 0", "0 -1 0", "0 2 -2", "-4 0 1", "-4 0 -4", "0 -4 0 -4 0", "-1 0 4 0 2", "-2 2 0", "1 0 -4 0", "3 -2 2", "0 2 3 -2", "2 -1 0 2 -1", "2 -1 -3", "3 -2 0 -4", "0 -3 4 -3 0", "-1 1 -1 0 -1", "0 -4 1 0", "-1 0 2", "4 0 2", "0 2 0", "0 1 0", "0 -4 0", "0 -2 0", "0 2 -2", "2 -2 0", "0 4 0", "0 3 0", "0 2 -2 0", "0 -1 0", "0 -3 0", "-4 0 -2", "-2 0 2", "1 0 4", "-2 0 -4", "0 3 -2", "3 -2 0", "1 -1 0", "-2 3 0", "0 -1 2", "0 -3 4", "4 -3 0", "-2 0 4", "0 4 -3", "-2 0 -4 0", "-2 2 -2", "3 0 1", "4 0 2", "-1 0 -1", "0 -2 3", "1 0 -4", "-1 0 -1 0", "-2 0 -3", "1 0 -3", "-2 0 3", "2 0 -2", "-2 2 -2 0", "-4 0 -2 0", "0 1 0 4", "0 3 -3", "2 0 1", "1 -4 0", "0 -4 1", "0 3 -2 0", "-3 4 0", "0 -4 0 -2", "2 -1 0", "0 3 0 1", "0 1 -4 0", "3 0 2", "-3 0 -4", "-4 0 2 -2 0", "0 -4 0 2 -2", "2 0 -2 0", "0 4 -3 0", "-4 0 2", "-4 0 2 -2", "-2 2 0", "-4 1 0", "0 4 -4", "-2 0 2 0", "0 -2 0 2", "1 0 3", "-2 0 4 0", "2 0 -4", "-2 3 -2", "0 2 0 1", "0 4 0 2", "0 2 -2 2", "0 1 -1", "0 -4 0 -3", "-1 0 -4", "-1 0 -2", "2 -2 0 -4 0", "2 0 3", "0 -4 0 2", "0 -3 4 0", "0 3 -3 0", "0 -4 0 -2 0", "-2 0 -2", "0 -3 3", "0 -2 0 -4", "0 -4 1 0", "4 0 2 -2", "-3 0 -4 0", "0 -3 4 -3 0", "2 -2 0 2", "0 1 0 -1", "2 -2 0 4 0", "2 -2 0 4", "1 0 -4 0", "-3 0 3 0", "0 3 0 -2", "2 -2 3", "0 2 0 -2 0", "0 1 0 3", "1 0 4 0", "-4 4 -4 0", "-2 0 1", "0 -4 0 3 0", "1 0 1 0", "-1 0 3", "0 -1 2 -1", "0 -1 0 -1", "0 4 0 3", "0 -2 0 4", "0 -4 4", "0 3 0 1 0", "1 0 -3 3", "0 2 -1", "-1 0 1", "-2 0 -3 0", "1 -1 0 -2", "-1 0 -2 0", "3 0 3", "-1 1 0", "3 0 -2", "3 0 4 0", "0 2 -2 2 -2 0", "0 1 0 -4", "0 2 0 4 -3", "-2 0 -2 0", "0 3 0 -2 0", "-2 0 -2 3", "0 2 0 3", "0 -2 0 2 0", "0 -3 3 0", "4 0 -3", "0 1 0 -3", "1 0 4 -3 0", "2 -2 0 -2", "0 -1 1", "-1 1 -1 0", "0 1 0 -1 1", "0 -3 0 -3", "-1 0 -3", "4 -3 0 1", "-3 4 0 2", "0 2 -2 0 -3 4", "3 -2 0 -3 0", "0 -2 0 3", "-2 0 -4 0 2", "0 2 -2 0 -4 0", "0 -2 0 4 0 3", "4 0 -2 0", "0 -4 0 -3 4", "0 1 0 -4 0", "0 -2 2", "0 4 0 4", "2 0 -4 0", "-4 0 -1 2", "3 0 3 0", "0 3 0 2", "0 2 -1 0", "2 -2 3 0", "0 1 -1 0", "0 1 0 4 0", "0 1 -4 0 -2", "0 -2 0 2 -2 0", "0 -2 0 -3", "-4 0 1", "-2 0 2 -2 0 3 0", "-2 0 3 0 1 -4 0", "4 -1 0", "0 2 -2 0 2", "2 0 2 -2", "1 0 -4 4", "-1 0 4", "2 -1 0 -4 0 -3", "0 -1 2 -1 0", "-1 0 3 0", "-3 0 3 0 1 0", "1 -4 0 -4", "0 1 0 -2", "-2 0 -4 0 3 0", "0 4 0 2 -2 2 -2 0 -4 0 3", "0 2 -2 0 4", "-2 0 2 -2 0", "0 -1 1 0", "1 -1 0 -2 0", "0 -4 0 3", "4 0 1", "-2 0 -1", "-1 0 -1 0 -1", "0 1 0 3 0", "-1 2 0", "-1 0 1 0", "3 -2 3", "0 -2 3 0", "3 0 2 0", "0 3 0 4 0", "-1 0 2", "0 -3 0 -1 0", "-4 0 -3", "-1 0 -2 3", "0 -2 3 -2", "0 -2 3 -2 0", "-2 0 -4 0 3", "0 3 0 3", "0 -2 0 -4 0", "0 4 0 -4 0", "1 0 2", "3 0 -2 3 -2", "-3 0 2 -2 0", "4 -3 0 2", "-3 0 -2 0", "2 0 4", "0 2 0 4", "2 0 4 -3", "0 2 0 4 -3 0", "-3 0 2", "-3 0 -3", "4 0 4", "1 0 -2", "-2 0 2 -2", "1 0 1", "2 0 4 -3 0", "-3 0 3", "3 -3 0", "0 3 0", "-3 3 -3 0", "-3 3 -3", "0 -3 3 -3", "0 -3 3 -3 0", "2 -1 0", "0 -3 3", "-3 0 -3", "3 -3 0 -3", "-3 0 -3 3", "0 2 -1", "0 1 0", "0 3 0 3", "0 -1 0", "3 -3 0 -3 3", "0 2 -1 0", "0 4 0", "0 3 -2", "-1 0 2", "3 -2 0", "0 -4 0", "0 -3 0", "3 0 2", "0 3 -3", "0 -3 4", "-3 0 -3 3 -3", "0 3 -2 0", "-1 0 4", "-1 0 3", "-1 0 3 0", "0 1 0 3 0", "1 0 -1", "0 1 0 -1 0", "3 0 1", "0 2 0", "0 -1 2 0", "-3 0 -2", "3 0 -3", "0 -2 3", "0 -3 3 -3 0 -3 3", "3 0 3", "0 2 -1 0 2", "0 2 -2", "2 -2 3", "1 -1 0 3", "0 3 -2 0 1 0", "0 4 0 -1", "0 1 -4", "2 -1 0 4", "0 4 -4", "0 1 0 3 0 1 0", "1 0 3", "0 1 0 3", "1 0 3 0", "2 0 -1", "0 -1 0 3 0 3 0", "0 2 0 3 0", "2 0 4 0 2", "-4 0 -3", "4 -4 0", "0 3 0 3 -3", "-4 0 3 0", "0 -3 4 -3", "-3 3 0", "-2 0 3", "0 -2 0", "1 0 -3", "2 -2 0", "3 0 -3 4", "-3 0 -3 3 -3 0", "3 -3 0 -3 3 -3 0", "0 -3 3 -3 0 -3 3 -3 0", "0 3 0 -3", "-3 3 -3 0 -3", "0 -3 3 -3 0 -3", "-3 3 -3 0 -3 3", "2 -1 0 2", "3 0 3 0", "2 0 3", "3 -3 0 -3 3 -3", "0 3 0", "0 2 0", "0 4 0", "0 -3 4", "0 1 0", "2 -1 0", "0 -1 0", "0 -3 3", "2 0 3", "0 4 -4", "1 -1 0", "0 3 -2", "3 0 3", "0 2 -1", "-4 0 -3", "0 -3 0", "-1 0 4", "-1 0 2", "4 -4 1", "4 -4 0", "0 -2 3", "3 -3 0", "0 1 -1", "0 1 -4 0", "3 0 3 0", "1 -4 0", "0 2 0 3", "3 -2 0", "0 3 0 3", "-1 0 3", "1 -1 0 4", "0 2 -1 0", "0 -3 4 -4", "3 0 1", "0 -2 0", "0 4 -4 0", "0 3 0 3 0", "1 0 3 0", "3 -2 2", "-4 0 -3 3", "3 0 -3", "0 -3 3 -3 0", "3 0 -2", "-4 1 0", "0 -4 4", "2 -1 0 -3", "0 3 0 1", "2 0 -3", "-3 0 1", "-4 1 -1", "0 2 -2", "-2 3 0", "1 0 1", "0 -1 0 2", "0 3 -2 2", "0 1 0 3", "0 -4 1", "0 -3 3 0", "-2 2 0", "-2 0 3", "1 0 4 0", "4 -4 1 0", "0 1 -1 2", "1 0 1 0", "0 1 0 1", "-1 0 4 -4", "2 -1 0 3", "1 -1 2", "-1 2 -1 0", "0 4 -4 1 -1", "0 -3 4 -4 1", "4 -4 0 -3 3", "0 -4 4 -4", "-1 0 2 -1", "-2 0 -1", "1 -1 0 4 -4", "0 4 0 3", "2 0 4", "4 -4 0 -3", "0 3 0 -2", "0 -3 4 0", "1 0 3", "-4 0 3", "-3 0 2", "0 3 -2 3", "0 2 0 3 0", "0 4 0 2", "4 -3 0", "-3 0 1 0", "0 2 0 -3", "0 1 0 3 0", "0 -4 0", "0 -4 0 -3", "2 -2 0", "2 0 -2", "0 3 -3", "2 -1 0 -3 4", "-1 0 -2", "1 -1 0 3", "-1 0 3 0", "0 -1 2", "0 -3 4 -4 1 0", "0 4 0 -1", "1 0 -3", "0 3 -2 0", "0 1 0 4 0", "0 4 0 -4", "0 4 0 3 -2", "3 -2 0 1 0", "2 -1 0 -3 0", "-3 0 -4", "0 4 -4 1 -1 0", "-1 0 4 -4 0", "0 4 -4 0 2", "-3 0 -1", "0 3 0 1 -1", "-1 0 4 0", "0 1 -1 2 -1 0", "2 -1 0 2", "0 2 0 -1", "-1 0 -1 0", "-1 0 2 -1 0", "0 1 0 2", "0 2 0 -3 4 -4", "1 0 3 0 2", "0 -2 3 -2", "3 -2 0 -1", "0 4 -4 0 -3", "1 0 -4", "-4 0 -3 3 -3 0", "-2 3 -2 0", "-2 3 -2", "0 4 0 2 0", "-4 0 3 0", "0 1 -4", "0 -3 3 0 -2", "0 -2 0 2", "-2 0 2 0", "3 0 -2 0", "-4 0 -3 0", "0 -3 0 3", "0 3 -3 0", "0 -3 4 -3 0 1 0", "0 3 -2 2 0", "2 0 2", "0 2 0 2 0", "0 3 0 -3", "3 0 -3 4", "0 1 0 1 0", "0 -3 3 -2 0 3", "0 -3 4 -4 0 -3 3 -2", "0 -3 0 2 0", "0 2 -2 0", "0 -3 3 -2", "2 0 -4 0 -3 3", "3 0 -2 3", "0 2 0 -2", "0 2 0 4 0", "-2 0 -2 3 0", "0 1 0 3 0 -2", "-3 3 -3", "0 -3 3 -3", "-3 3 -3 0", "1 0 4", "-4 0 2", "-1 0 -1", "3 0 2", "-3 4 -4", "4 0 3", "-2 0 2", "2 0 3 0", "0 2 -1 0 3", "-3 3 -2", "0 -1 0", "0 3 0", "-1 0 3", "0 3 -2", "-1 0 3 0", "0 1 0", "0 3 0 -1", "-1 0 -1", "3 0 -1", "0 -1 0 3", "-1 1 0", "-1 0 3 -2", "-1 0 -1 0", "0 -1 1 0", "0 -1 0 -1", "0 -1 1", "3 -3 0", "0 1 -1", "0 3 -3", "0 -1 0 -1 0", "0 -3 3", "0 -3 3 0", "0 3 0 3", "1 0 -1", "0 1 -1 0 3", "0 3 0 -1 1 0", "2 -1 0", "1 0 3", "0 3 -2 0", "0 3 -3 0", "0 -1 0 1", "0 2 -1 0", "-1 2 0", "0 1 0 -1", "1 0 -1 0", "0 -1 0 3 0", "0 -1 0 3 -2", "-2 2 0", "2 0 -2", "-1 0 3 -2 3 0", "0 -1 0 -1 0 3", "-1 0 3 -2 3", "-1 0 -1 0 3 -2", "0 2 0", "0 -3 0", "0 -1 2 0", "0 -1 0 -1 1 0 3", "0 -1 0 1 -1 0 3 -2", "1 -1 0 3 -2 3", "2 0 3", "0 3 -3 0 3", "0 -3 3 0 1 0", "1 -1 1 0", "0 3 -2 2 0", "3 0 3", "1 0 -3", "-1 1 0 1", "3 0 1 0 3", "0 -1 0 2 -1 0", "-1 0 -3 3 0", "3 0 1", "3 0 1 0", "0 -2 2", "-1 0 3 0 -1", "0 3 -2 0 -1 0", "3 0 -1 1", "1 -1 0 3 -2", "-1 0 3 -2 0", "0 3 0 -1 1", "3 0 -1 1 0", "-2 -1 0", "-1 0 -1 0 3", "0 -4 0 1 0", "3 0 -1 0", "3 0 -1 0 3", "1 -1 0 3", "1 0 3 0", "0 3 -2 0 1", "0 1 0 -1 0", "0 1 -1 0 3 0", "3 -2 0", "-1 0 1", "1 0 1", "1 -1 0", "0 -1 0", "-1 0 -1", "0 -1 0 -1", "1 -1 0", "0 1 0", "-1 0 3", "2 -1 0", "0 3 0", "0 -1 1", "-1 0 -2", "-2 2 -2", "-1 0 -1 0", "3 -3 0", "0 -2 0", "0 1 -1 0", "-2 0 -1", "0 3 -2", "-2 0 -1 0", "4 -3 0", "0 -1 1 -1 0", "0 -1 0 -1 0", "0 -1 0 3", "-3 0 1", "-1 0 3 0", "3 0 -1", "2 0 3", "0 2 0", "-1 0 -3", "0 -2 3", "0 -1 0 -2", "0 -1 0 -1 1", "0 2 -1", "-1 0 3 -2", "0 1 0 3", "-2 2 -1 0", "2 0 -1", "3 -3 0 1", "-1 0 1 0", "-2 2 0", "3 -2 0 -1 0", "-1 0 2", "0 2 -1 0", "1 0 1", "0 -4 0", "0 4 -3", "0 4 -3 0", "0 -1 0 -3", "0 -3 3 -3 0", "-2 2 -2 0", "-3 0 4", "0 3 -2 0 -1 0", "0 1 0 3 0", "0 3 -3 0", "2 -1 0 2", "-1 0 2 -1", "1 -1 0 -2", "-1 0 1", "3 -2 2", "0 -1 1 0", "-1 0 -2 2", "0 3 0 -1", "-3 0 1 0", "0 -1 0 3 0", "2 -2 0", "0 -3 0", "0 2 0 3", "3 -3 0 1 0", "1 0 -2", "-2 3 0", "-2 0 -2", "2 0 -1 0", "0 -1 0 1", "0 -1 2", "2 0 3 0", "3 0 -2", "0 2 0 -1", "-3 0 2", "-1 0 -2 3", "3 0 -1 1", "3 0 -1 1 -1 0", "0 2 3", "1 -1 0 3", "3 -2 2 -1 0", "-2 2 -2 2", "0 -1 0 -2 2", "-1 0 -1 0 -1", "0 -1 0 -1 1 -1 0", "2 -2 3", "-1 0 -1 0 -2", "-1 0 -2 0", "3 0 1", "0 3 0 1", "-1 0 3 -2 0 -1 0", "0 3 -2 2 -1 0", "0 1 0 -1 0", "3 0 1 0", "2 -1 0 -1", "0 -2 0 -1", "0 1 -1 0 -2 3", "-4 0 1", "0 2 0 -1 0", "-1 0 3 0 -1", "3 0 -1 0", "0 3 0 3", "3 -3 0 2", "-3 0 1 0 1", "0 3 0 -3", "-3 0 3", "4 -3 0 3", "-2 2 -2 0 -2", "2 -2 0 -2 0", "-1 0 -3 3 -3 0", "1 -1 0 -3", "0 -1 0 1 0", "0 -3 -2 3 -3 0", "-2 0 2 0 3 0", "3 0 -2 0", "0 -2 0 1", "0 -1 0 -3 0", "0 3 0 -1 1 -1 0", "-2 2 0 -1", "2 0 -1 1", "3 -2 0 -1 0 -3", "0 3 -3 0 1 0", "0 -3 3 -3 0 1", "0 -2 3 0", "2 -2 0 -2", "-3 0 1 -1 0", "-1 2 0 3", "0 -1 0 -1 1 -1 0 -2 0", "-2 2 -1 0 3", "-2 2 -1 0 3 -2", "2 3 0", "0 -1 0 2", "-1 3 0", "3 0 2", "3 -1 3", "-2 3 0 -1 1", "-2 3 0 -1", "0 -1 0 -1 0 -2", "0 -4 1", "-4 1 0", "0 -1 1 0 -2 0", "0 -2 3 -2 2", "3 -2 2 -1 0 3", "2 -2 3 0 -1", "1 -1 0 -1 0", "1 0 2", "-1 0 -4", "2 -1 0 -1 0", "-1 0 -1 1", "0 3 -2 0 -1 0 -1 0", "1 -1 0 3 -2 0 -1 0 -1", "0 -1 0 -1 0 -1 1", "0 1 0 3 -2", "0 -1 0 -1 1 0", "0 -1 0 3 -2 2 -1 0", "1 0 1 -1 0", "3 -2 0", "3 -2 0 -1", "-2 0 -1 0 3", "0 1 -1", "0 3 0 1 0", "3 0 -3", "2 -2 2", "-2 0 -1 0 -1", "3 -2 0 -1 0 -1", "0 -2 2", "0 3 -2 0", "0 3 -2 0 -1", "1 0 3", "-1 1 0"]
  out "Numeric":i32
  in  "subarray 3":string[](array[string])=array[8497 elements]
  out "sum":i32
  in  "subarray":string[](array[string])=array[4675 elements]
  in  "List of common substrings and the number of times they occur":string[][](array[string])
  in  "Array 4":u32[](array[colorbox])=[16448250, 11461119, 4390369, 3473009, 720406, 188173, 15137024, 16765472, 16350208, 16714500, 9895940]
  in  "Boolean":bool
  out "Array 2":u32[][][](array[colorbox])=[[[16448250, 6878717, 243648, 2448086, 215036, 7470158, 1425154, 15857665, 16566787, 16714500, 9895940]]]
  out "Array":dbl[][][](array[numeric])
  out "Number of elements in clusters":i32[](array[numeric])
  out "Weighted array of NEW cluster centers":dbl[][][](array[numeric])
  out "Clusters":string[][](array[string])
  out "Weighted arrays for movement patterns":dbl[][][](array[numeric])
  in  "milliseconds to wait":u32
  out "Weighted arrays of cluster centers":dbl[][][](array[numeric])
  in  "Cluster centers":string[](array[string])=["1 0 1 0 1 0 1 0", "2 0 2 0 2 0 2 0", "3 0 3 0 3 0 3 0", "4 0 4 0 4 0 4 0", "1 0 4 0 1 0 4 0", "2 0 3 0 2 0 3 0", "1 0 2 0 1 0 2 0", "3 0 4 0 3 0 4 0", "1 0 3 0 1 0 3 0", "2 0 4 0 2 0 4 0"]
  in  "Full transition sequence from service to end":string[](array[string])=["-2 0 3 0 -3 0 4 -4 0\r\n", "0 3\r\n", "0 4 -3 0 -4 1 0 4 -3 0\r\n", "0\r\n", "-2 0 3 -3 0 -4 1 -4 0 3 -3 4 -3 0 2 0 3\r\n", "0 3 0 1\r\n", "0 1 0 3\r\n", "0 3 -2 0 4\r\n", "0\r\n", "0 -3 4 0 2 -2 0 -3 0 3 -2 3 -3 4\r\n", "0 -3 4 -3 0\r\n", "-2 0 -2 2 0\r\n", "0 3 -2\r\n", "0 4 -3 0 3 -2 0 -3 4 -3 0 3 -2 2 -2 0 4 0\r\n", "2 0 1 -4 0 3 0 -4 4 0 -4 4 0 2 0 4 0 -3 4 -3 0 -4 0 4\r\n", "0 4\r\n", "-2 0 -2 0 3 0\r\n", "0 3 0 -2 3\r\n", "0 4 0 4 -4 0 2 0 -4 4 -3 0 -2 2 -2 0 4 -3 0 2 0 3 0\r\n", "0 4 -3 0 1 -1 0 3 0 -2 2 -2 0 -3 4 -3 0 4 -4 1 0\r\n", "", "0 -3\r\n", "2 0 3 0 1 0 -2 3\r\n", "0\r\n", "1 -1 0\r\n", "0 -2 3 0\r\n", "0 1 0 4 0 4 -4 4\r\n", "0 1 -1 0 3\r\n", "0 2 -2 3 -3 4\r\n", "-2 2 0 -2 3\r\n", "0 -1\r\n", "0 4 -4 4 0 3 0 -2 0 -4 0 1 -4\r\n", "-2 0 4 0 -3 3 0 -2 2 -2 0 -4 0 4 0\r\n", "0 -1 0 -4 4 -4 1 -4 0\r\n", "1 -4 1 0 2 0 -3 0 2 0 -2 0 1 0 1 -4 4 -4 1 0 3 -2 0 -4 4 -4\r\n", "0 1 -4 4 -4 1\r\n", "0 3 0 -3 3 0 1 0 1 -4 4\r\n", "0 1 -4 0 1 -4\r\n", "0 3 -2 0 1 -4 1 0 2 0 4 0 4 0 -1 2 -1 0\r\n", "1 0 -1 0 2 0 4 -4\r\n", "-4\r\n", "-1 0 4\r\n", "0 1 -1 0 1 -4 0\r\n", "-1 0 1 -4 0 3 0 2 0 4 0 -4 4 -4 0 -1 0 -4 0 -2 0 4\r\n", "0 4 0\r\n", "0 4 -4 0 2 -1 0 2 0 4 -4 1 -4 4 0 3\r\n", "0 4 0 2 0\r\n", "1 0 -1 1 0 -4 1 -4 1 0 -4\r\n", "0 3 -2 0 -4\r\n", "2 -1 0 -4 4 -4 0 2 0 4\r\n", "1 0\r\n", "-1 0 -1 1 0 -4\r\n", "0 3 0\r\n", "0 -4 4 -4 0 -4 0 4 0 2 0 1 -4 4\r\n", "-1 0 1 -4\r\n", "-1 0 2 -1 0 2\r\n", "1 -1 0 4 -4 1\r\n", "-1 0 1 -4 4 -4 0 -4 4\r\n", "0 3 0 3 0 1 -1 0 1\r\n", "-1 0 4 0 4 -4 1 0 -4 0\r\n", "1 0 4\r\n", "0 -1 0 2 -1 0 -2 3 -2 0 -4 4 -4\r\n", "0 3 0\r\n", "2 -1 0 1 -4 4 -4 0 2 0\r\n", "0 4 -4 1 0 1 0 1 -4 0 2 0 4 0 4 -4 1\r\n", "1 -1 0 3 0 3 0 1 0 4\r\n", "0 -4 0 -2 0 -4\r\n", "0 -4 4 -4 0 -2 0 2 0\r\n", "-1 0 4 -4 0\r\n", "1 0 -1 2 0 4\r\n", "0 2 0 -2 0\r\n", "0 1 -4 0 -4 0 3 -2 0 -4 0 -4 4 -4 1\r\n", "0 4 0 4 0 4 0 4 0 -2 3 0 3 0 4 0\r\n", "-4 -1\r\n", "-2 0 1 0 -4 4\r\n", "0 4\r\n", "-2 2 0 -1 -4 1 0 3 0\r\n", "-1 0 -1 2\r\n", "0 -1 1 0 4 0 3 -2 0 -2 3 -2 0 4 0 -2 2\r\n", "2 -1 0 4\r\n", "0 4 0 2 0 -2 0\r\n", "1 -1 0 3 0 -4 4 -4 0\r\n", "2 -1 0 3 -2 0 -3 0 3 0 -3 0\r\n", "0 4 0 4 -4 1 -1 0 -3 0 1 -4 1 0 4 0 -4 0 -4 4 -4 1\r\n", "0 -4 1 0 -4 4\r\n", "0 4 0 -2 2 -2 2 -2 2\r\n", "-2 2 -1 0 4 0 2 0 4 0 2 -2 0 4\r\n", "1 0 -1 0 -1 0 1 -1\r\n", "-2 2 -2 3\r\n", "1 0 -1 0 -1 2 0 2 -2 0 -4 0\r\n", "-2 2 0 3 -2 2\r\n", "0\r\n", "1 -1 0 3\r\n", "0 4 0\r\n", "-2 0 1 -4 0 -3 0\r\n", "1 0 -1 2 -1 1 -4\r\n", "0 4\r\n", "-2 0 -1 1\r\n", "0 3 0 3 0 3 -2\r\n", "-4 0 -4 4\r\n", "0 4 0 -4 0 -4\r\n", "-2 2 0 4 -4 0 2 -2\r\n", "-2 2 -2 0 -1\r\n", "0 4 -3 0\r\n", "0 1 0 -1 1\r\n", "-4 0\r\n", "-2 0 3 0 1 0 3 -2 0 -1 0 4 0 3 0 -3 3 -3\r\n", "0 4 0 -2 0 1 0 -4 4 -3 0 1 0 4 0 -4 1 0 3 -3 0\r\n", "0 -1 2\r\n", "2 0 -3 4 0\r\n", "-4 0 -3 3 -3 0 -3 3 0 -2 3 0\r\n", "0 -1 1 -4 4 -3 0 3 0\r\n", "0 -1 2 0 3 0 1 -4 4 0 2 0\r\n", "2 -2 0 -4 0 -4 4 0 -4\r\n", "1 -1 2 -1\r\n", "2 0 -2 0 4 0 2 0 3 0 -2 0 -4\r\n", "1 -1 0 -1\r\n", "0 1 -4 1\r\n", "0 4 0 -1 1 -1 0\r\n", "0 3\r\n", "-2 0\r\n", "1 -4 0 -2 0 4 0 -4 0 4 -3 0 1 -4 0 1\r\n", "0 -3 3 -2 0 3 0 -2 2\r\n", "1 0\r\n", "2\r\n", "0 -4\r\n", "0 4 0 -4 0 -3 3 -3 0 -2 0 -2 0 4 0 -1 1 0 3 0 -4 1 -4 0 4\r\n", "2 0 -1 1\r\n", "0 2 0 4 0 4 -4 0 -1 2\r\n", "0 3 -2 0 3 -2\r\n", "1 0 -3 3 0 -4\r\n", "0 -3 3 0 -1 0\r\n", "2 -2 0 1\r\n", "-4 1 -4 1 -4 0\r\n", "0 4 0 2 0 -4 1 2 -1 0 4 0 1 0 4 -4 4 0 -4 4 0\r\n", "-2 0 3 0 -2 0\r\n"]
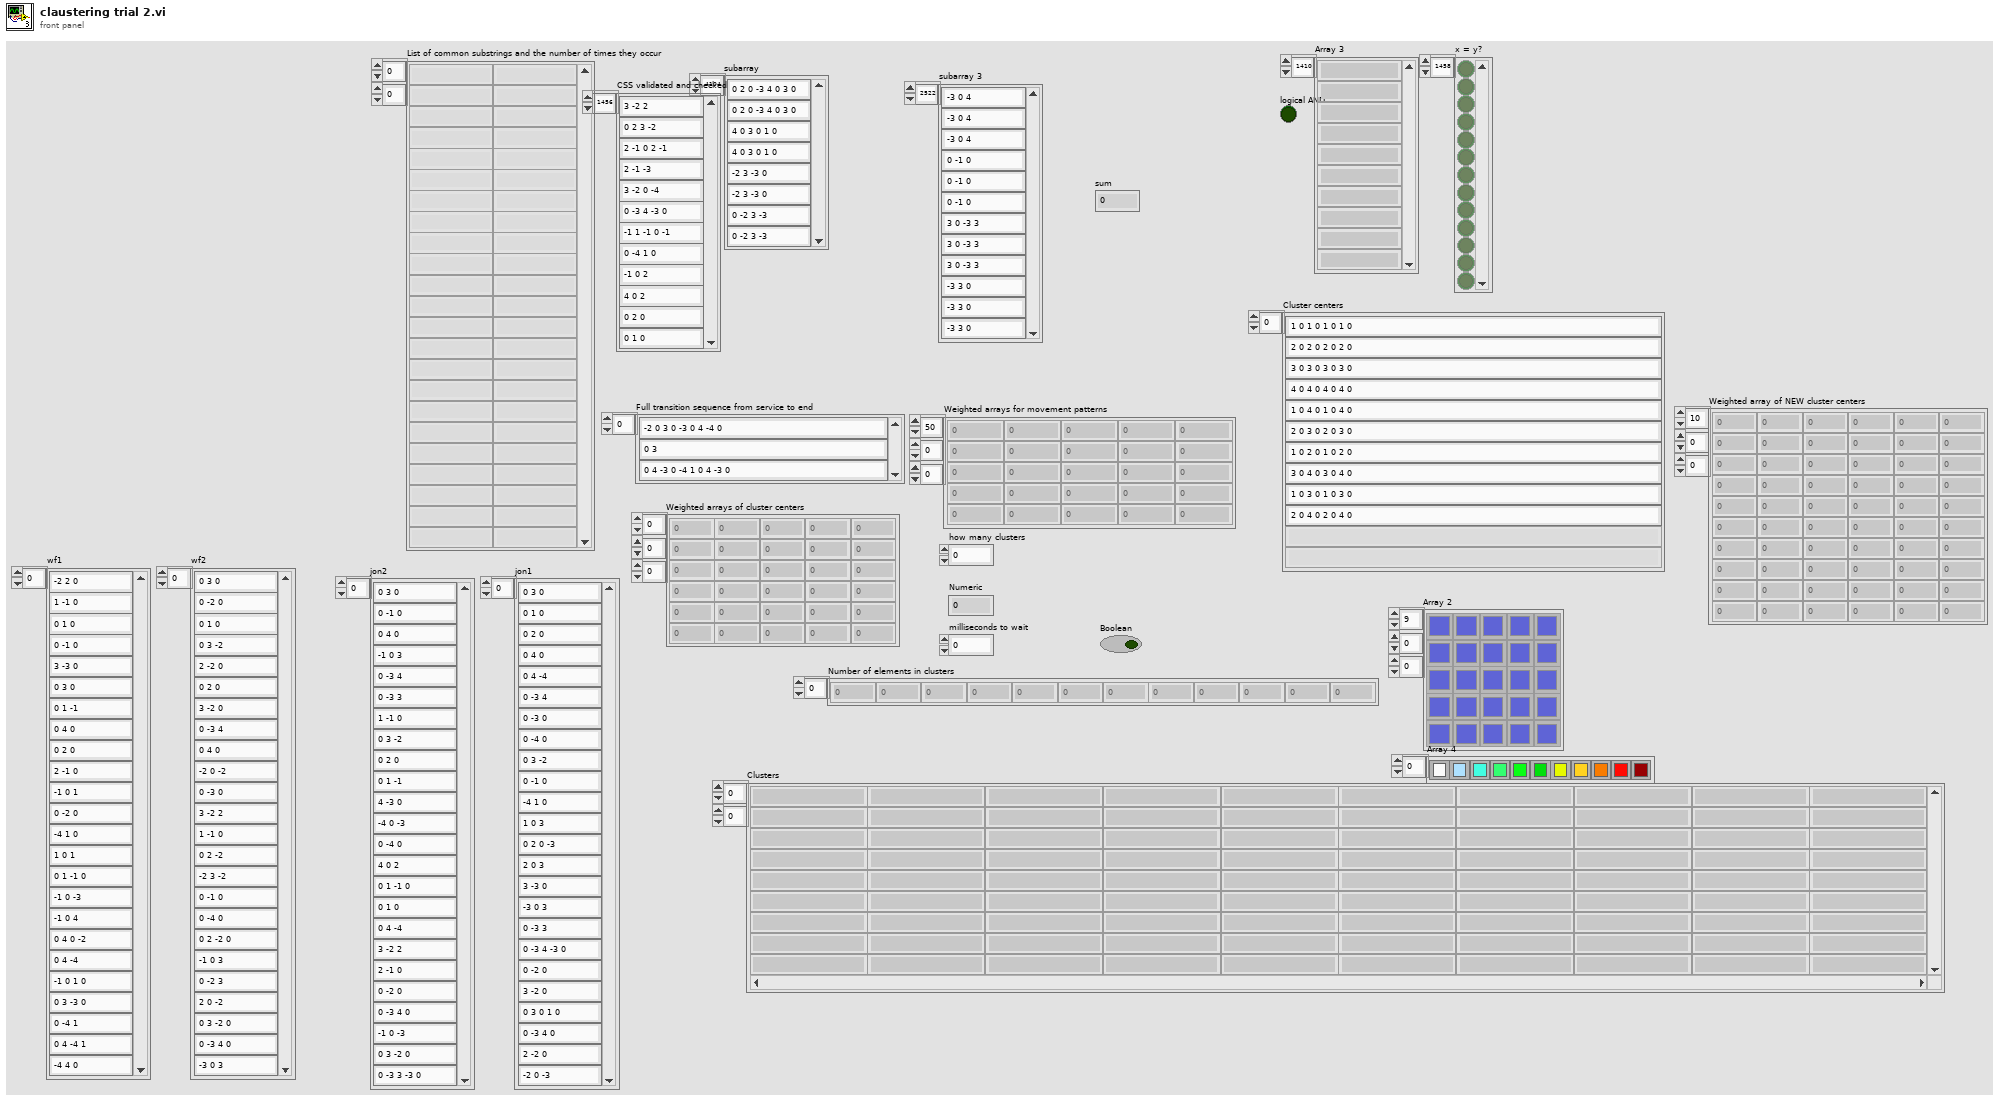
[diagram p1: front panel]
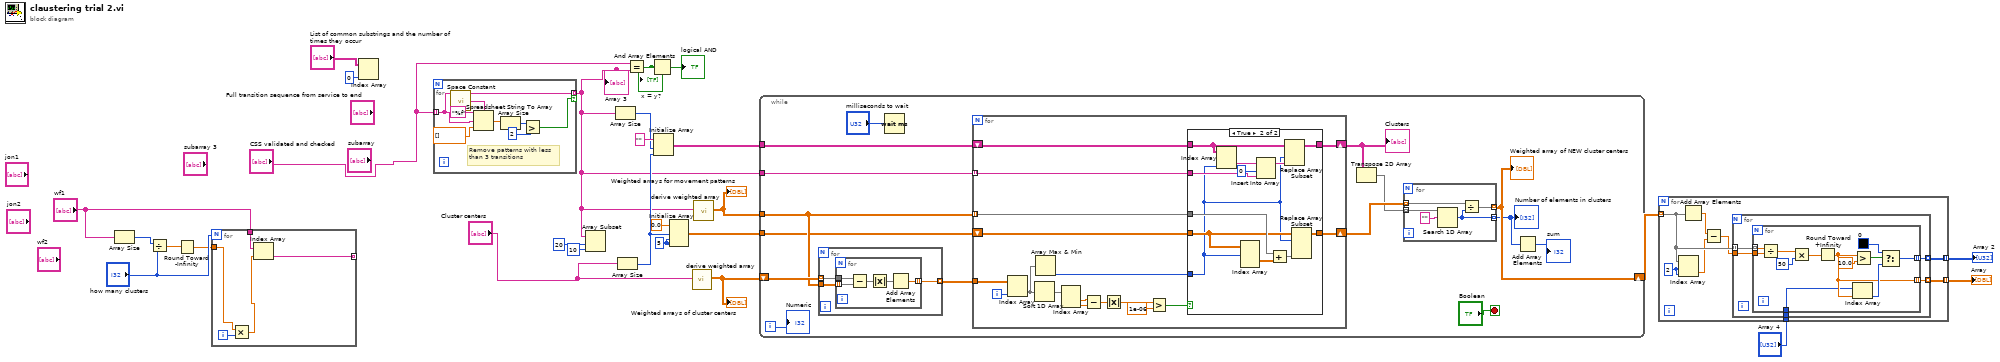
[diagram p0: block diagram]
diagram:
  w24 = 5 ("dimension size")
  n1 = Array Size(array="wf1") -> (size(s)=w12:i32)
  n2 = Divide(x=w12, y="how many clusters") -> (x/y=w11:dbl)
  n3 = Round Toward -Infinity(1:w11) -> (0:w9:dbl)
  n4 = for {
    N: "how many clusters" -> [_]
    tunnel: w9 -> [w31]
    tunnel: "wf1" -> [w29]
    tunnel: [w28] -> _ mode=indexing
    i -> [w32]
    n5 = Multiply(x=w31, y=w32) -> (x*y=w30:dbl)
    n6 = Index Array(array=w29, index=w30) -> (element=w28:string)
  }
  n7 = Index Array(array="List of common substrings and the number of times they occur", index (col)=0 ("disabled index (col)")) -> ()  [unwired: 1 in, 1 out]
  n8 = for {
    tunnel: "CSS validated and checked" -> [w34] mode=indexing
    tunnel: [w34] -> w4 mode=indexing if=w33
    # "Remove patterns with less \nthan 3 transitions"
    n9 = call <vilib>:"Space Constant.vi"() -> ("String"=w39:string)
    n10 = Spreadsheet String To Array(delimiter (Tab)=w39, format string="%f", spreadsheet string=w34, array type (2D Dbl)=dbl[] [] ("array 2")) -> (array=w37:dbl[])
    n11 = Array Size(array=w37) -> (size(s)=w36:i32)
    n12 = Greater?(x=w36, y=2) -> (0:w33:bool)
  }
  "Array 3" <- w4
  n13 = Array Subset(array=w4, index=20, length=10) -> ()  [unwired: 1 out]
  n14 = Array Size(array=w4) -> (size(s)=w26:i32)
  n15 = Array Size(array="Cluster centers") -> (size(s)=w23:i32)
  n16 = Equal?(x="CSS validated and checked", y=w4) -> (x = y?=w6:bool[])
  "x = y?" <- w6
  n17 = And Array Elements(Boolean array=w6) -> (logical AND=→"logical AND":bool)
  n18 = Initialize Array("" ("spreadsheet string"), w26, w23) -> (w13:string[][])
  n19 = Initialize Array(0.0, w23, w24, w24) -> (w22:dbl[][][])
  n20 = call "derive weighted array.vi"("Full transition sequence from service to end"="Cluster centers") -> ("Weighted arrays"=w1:dbl[][][])  [unwired: 10 in]
  "Weighted arrays of cluster centers" <- w1
  n21 = call "derive weighted array.vi"("Full transition sequence from service to end"=w4) -> ("Weighted arrays"=w3:dbl[][][])  [unwired: 10 in]
  "Weighted arrays for movement patterns" <- w3
  n22 = while {
    tunnel: w4 -> [w50]
    shift-right: [w44] -> w19
    shift-left: w1 -> [w55]
    tunnel: w3 -> [w54]
    tunnel: w13 -> [w49]
    tunnel: w22 -> [w48]
    i -> [w41]
    stop <- "Boolean" stop-if-true
    n23 = for {
      tunnel: w55 -> [w94] mode=indexing
      tunnel: w54 -> [w93]
      tunnel: [w92] -> w53 mode=indexing
      n24 = for {
        tunnel: w94 -> [w99]
        tunnel: w93 -> [w98] mode=indexing
        tunnel: [w95] -> w92 mode=indexing
        n25 = Subtract(x=w99, y=w98) -> (x-y=w97:dbl[][])
        n26 = Absolute Value(x=w97) -> (abs(x)=w96:dbl[][])
        n27 = Add Array Elements(numeric array=w96) -> (sum=w95:dbl)
      }
    }
    n28 = Wait (ms)(milliseconds to wait="milliseconds to wait") -> ()  [unwired: 1 out]
    n29 = for {
      tunnel: w50 -> [w66] mode=indexing
      tunnel: w54 -> [w63] mode=indexing
      tunnel: w53 -> [w77]
      shift-right: [w65] -> w46
      shift-left: w49 -> [w67]
      shift-right: [w62] -> w47
      shift-left: w48 -> [w61]
      i -> [w70]
      n30 = Index Array(array=w77, index (col)=w70) -> (element=w69:dbl[])  [unwired: 1 in]
      n31 = Sort 1D Array(array=w69) -> (sorted array=w72:dbl[])
      n32 = Array Max & Min(array=w69) -> (min index (indices)=w68:i32)  [unwired: 3 out]
      n33 = Index Array(array=w72) -> (element #1=w76:dbl, element #2=w71:dbl)  [unwired: 2 in]
      n34 = Subtract(x=w76, y=w71) -> (x-y=w74:dbl)
      n35 = Absolute Value(x=w74) -> (abs(x)=w73:dbl)
      n36 = Greater?(x=w73, y=1e-06) -> (0:w64:bool)
      n37 = case shown="True" w64 {
        tunnel: w68 -> [_ w81]
        tunnel: w67 -> [w79 w89]
        tunnel: w66 -> [_ w90]
        tunnel: [w79 w87] -> w65
        tunnel: w63 -> [_ w84]
        tunnel: [w78 w80] -> w62
        tunnel: w61 -> [w78 w83]
        frame False {
        }
        frame True {
          n38 = Index Array(array=w89, index (col)=w81) -> (element=w91:string[])  [unwired: 1 in]
          n39 = Index Array(array=w83, index (dim 0)=w81) -> (element=w85:dbl[][])  [unwired: 2 in]
          n40 = Insert Into Array(array=w91, index=0, new element=w90) -> (w88:string[])
          n41 = Add(x=w84, y=w85) -> (x+y=w82:dbl[][])
          n42 = Replace Array Subset(array=w89, new element=w88, index (col)=w81) -> (w87:string[][])  [unwired: 1 in]
          n43 = Replace Array Subset(array=w83, new element=w82, index (dim 0)=w81) -> (w80:dbl[][][])  [unwired: 2 in]
        }
      }
    }
    "Clusters" <- w46
    n44 = Transpose 2D Array(2D array=w46) -> (transposed array=w45:string[][])
    n45 = for {
      tunnel: w47 -> [w58] mode=indexing
      tunnel: w45 -> [w60] mode=indexing
      tunnel: [w57] -> w44 mode=indexing
      tunnel: [w56] -> w43 mode=indexing
      n46 = Search 1D Array(1D array=w60, element="" ("spreadsheet string")) -> (index of element=w56:i32)  [unwired: 1 in]
      n47 = Divide(x=w58, y=w56) -> (x/y=w57:dbl[][])
    }
    "Weighted array of NEW cluster centers" <- w44
    "Number of elements in clusters" <- w43
    n48 = Add Array Elements(numeric array=w43) -> (sum=→"sum":i32)
    "Numeric" <- w41
  }
  n49 = for {
    tunnel: w19 -> [w107] mode=indexing
    tunnel: [w102] -> w20 mode=indexing
    tunnel: [w101] -> w21 mode=indexing
    tunnel: "Array 4" -> [w100]
    w106 = 2 ("index (row)")
    n50 = Index Array(array=w107, index (row)=w106, index (col)=w106) -> (element=w105:dbl)
    n51 = Add Array Elements(numeric array=w107) -> (sum=w104:dbl)
    n52 = Subtract(x=w104, y=w105) -> (x-y=w103:dbl)
    n53 = for {
      tunnel: w107 -> [w112] mode=indexing
      tunnel: w103 -> [w111]
      tunnel: [w110] -> w101 mode=indexing
      tunnel: [w109] -> w102 mode=indexing
      tunnel: w100 -> [w108]
      n54 = for {
        tunnel: w112 -> [w124] mode=indexing
        tunnel: w111 -> [w123]
        tunnel: [w114] -> w110 mode=indexing
        tunnel: [w115] -> w109 mode=indexing
        tunnel: w108 -> [w113]
        n55 = Divide(x=w124, y=w123) -> (x/y=w122:dbl)
        n56 = Multiply(x=w122, y=50) -> (x*y=w120:dbl)
        n57 = Round Toward +Infinity(x=w120) -> (ceil(x): smallest int >= x=w114:dbl)
        n58 = Index Array(array=w113, index=w114) -> (element=w116:u32)
        n59 = Greater?(x=w114, y=10.0) -> (0:w118:bool)
        n60 = Select(t=u32 0, s=w118, f=w116) -> (s? t:f=w115:u32)
      }
    }
  }
  "Array 2" <- w20
  "Array" <- w21
